vi "信息读取.vi"() -> ()   [LabVIEW 2018]
uses:
  <vilib>/addons/database/Connection.llb/DB Tools Open Connec (Path).vi
  <vilib>/addons/database/NI_Database_API.lvlib
panel:
  out "表格控件":string[][](table)
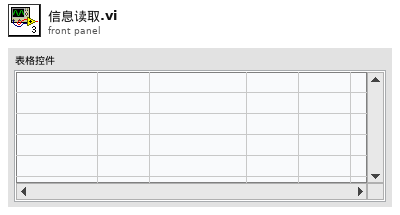
[diagram p1: front panel]
types:
  T1 = typedef "NI_Database_API.lvlib/Conn ObjectReference.ctl" = refnum<k1>
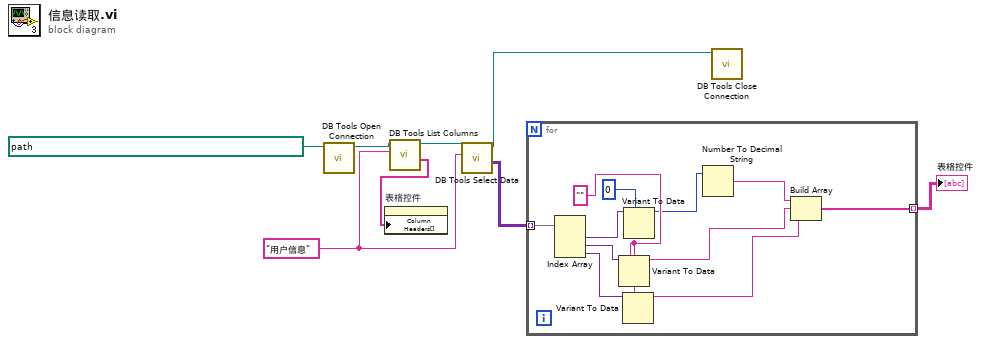
[diagram p0: block diagram]
diagram:
  w1 = "用户信息" ("table")
  n1 = call-poly <vilib>:"DB Tools Open Connection.vi"("connection information"=path "D:/SoftwareWS/LabVIEW/LV-DB/file/用户信息.udl") -> ("connection reference"=w5:T1)  [unwired: 7 in, 1 out]
  n2 = call <vilib>:"DB Tools List Columns.vi"("table"=w1, "connection reference"=w5) -> ("columns"=w2:string[], "connection reference out"=w4:T1)  [unwired: 2 in, 2 out]
  n3 = property on="表格控件" class="Tbl (严格)"("Column Headers[]"=w2) -> ()  [unwired: 2 in, 2 out]
  n4 = call <vilib>:"DB Tools Select Data.vi"("table"=w1, "connection reference"=w4) -> ("data"=w6:variant[][], "connection reference out"=w7:T1)  [unwired: 4 in, 1 out]
  n5 = for {
    tunnel: w6 -> [w19] mode=indexing
    tunnel: [w9] -> w3 mode=indexing
    w14 = ""
    n6 = Index Array(array=w19) -> (element #1=w18:variant, element #2=w16:variant, element #3=w15:variant)  [unwired: 3 in]
    n7 = Variant To Data(type=w14, Variant=w16) -> (data=w11:string)  [unwired: 1 in, 1 out]
    n8 = Variant To Data(type=w14, Variant=w15) -> (data=w10:string)  [unwired: 1 in, 1 out]
    n9 = Variant To Data(type=0, Variant=w18) -> (data=w13:i32)  [unwired: 1 in, 1 out]
    n10 = Number To Decimal String(number=w13) -> (decimal integer string=w12:string)  [unwired: 1 in]
    n11 = Build Array(w12, w11, w10) -> (w9:string[])
  }
  "表格控件" <- w3
  n12 = call <vilib>:"DB Tools Close Connection.vi"("connection reference"=w7) -> ()  [unwired: 6 in, 1 out]
